vi "Hardware Out - NI 9411-3 (Digital Input).vi"(11 "FPGA Ref":T1) -> ()   [LabVIEW 2015, in "ECS-RT.lvlib"]
uses:
  ECS-RT.lvlib
  Typedefs/FPGA Refs/Generic FPGA Ref.ctl
  <vilib>/Utility/error.llb/Error Cluster From Error Code.vi
  <vilib>/rvi/errors/niLvFpgaAdjustHostInterfaceError.vi
  <vilib>/rvi/interface/nirviReadWriteControl/nirviReadWriteControl.xnode
  <vilib>/rvi/interface/Simulation/niFpgaSimulationCallBeginRW.vi
  NiFpgaLv.dll
  ECS-Shared.lvlib
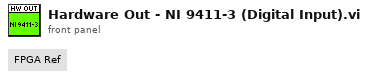
[diagram p1: front panel]
types:
  T1 = typedef "ECS-Shared.lvlib/Generic FPGA Ref.ctl" = refnum<k20>
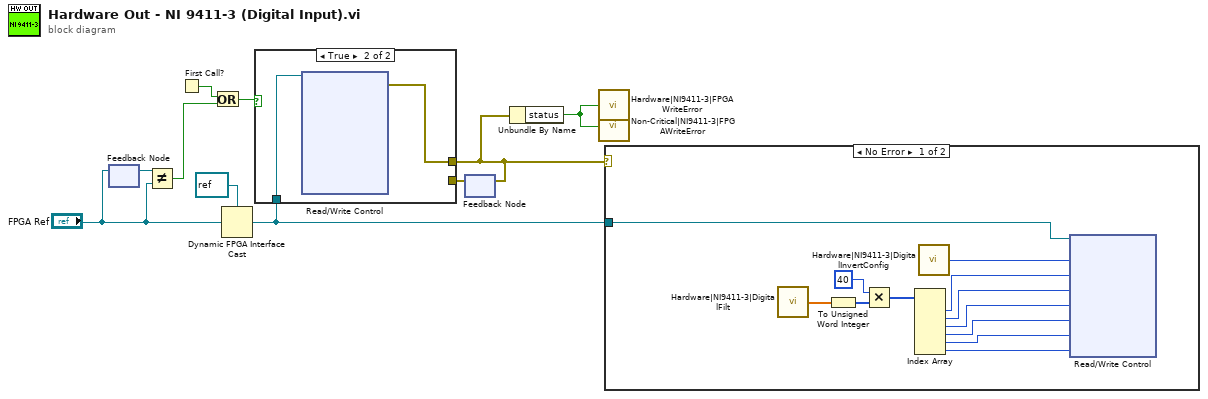
[diagram p0: block diagram]
diagram:
  n1 = feedback #1() -> (w6:T1)  [unwired: 1 in]
  n2 = feedback-in #1("FPGA Ref") -> ()
  n3 = Not Equal?(x=w6, y="FPGA Ref") -> (x != y?=w5:bool)
  n4 = First Call?() -> (First Call?: T/F=w7:bool)
  n5 = Or(x=w7, y=w5) -> (x .or. y?=w8:bool)
  n6 = Dynamic FPGA Interface Cast(Session In=refnum<k20> refnum ("NI 9411"), Type="FPGA Ref") -> (Session Out=w3:refnum<k20>)
  n7 = feedback #2() -> (w9:errorcluster)  [unwired: 1 in]
  n8 = case shown="True" w8 {
    tunnel: [w11 w12] -> w2
    tunnel: w9 -> [w11 _]
    tunnel: w3 -> [_ w13]
    frame False {
    }
    frame True {
      n9 = xnode "Read/Write Control"("FPGA VI Reference In"=w13) -> ("error out"=w12:errorcluster)  [unwired: 8 in, 1 out]
    }
  }
  n10 = feedback-in #2(w2) -> ()
  n11 = Unbundle By Name(w2) -> ("status"=w1:bool)
  n12 = call "Hardware|NI9411-3|FPGAWriteError"("Value"=w1) -> ()
  n13 = call "Non-Critical|NI9411-3|FPGAWriteError"("Fault"=w1) -> ()  [unwired: 2 in]
  n14 = case shown="No Error" w2 {
    tunnel: w3 -> [w21 _]
    frame No Error {
      n15 = call "Hardware|NI9411-3|DigitalFilt"() -> ("Value"=w25:sgl[])
      n16 = To Unsigned Word Integer(number=w25) -> (unsigned 16bit integer=w24:u16[])
      n17 = Multiply(x=u16 40 ("y"), y=w24) -> (x*y=w23:u16[])
      n18 = Index Array(array=w23) -> (element #1=w14:u16, element #2=w15:u16, element #3=w16:u16, element #4=w17:u16, element #5=w18:u16, element #6=w19:u16)  [unwired: 6 in]
      n19 = call "Hardware|NI9411-3|DigitalInvertConfig"() -> ("Value"=w20:u32)
      n20 = xnode "Read/Write Control"("FPGA VI Reference In"=w21, "9411-3.Invert"=w20, "9411-3.0.Filt"=w14, "9411-3.1.Filt"=w15, "9411-3.2.Filt"=w16, "9411-3.3.Filt"=w17, "9411-3.4.Filt"=w18, "9411-3.5.Filt"=w19) -> ()  [unwired: 1 in, 2 out]
    }
    frame Error {
    }
  }
